vi "Status.Simple LED Status Indicator.vi"(7 "Show OK Indication":bool, 8 "error in":errorcluster, 10 "Blink on Error":bool, 11 "LED Status":refnum<vi>) -> (0 "error out":errorcluster)   [LabVIEW 2024, in "EQMF.lvlib" / "Status Utils.lvlib"]
uses:
  Status Utils.lvlib
panel:
  out "LED Status":bool
  in  "Test":bool
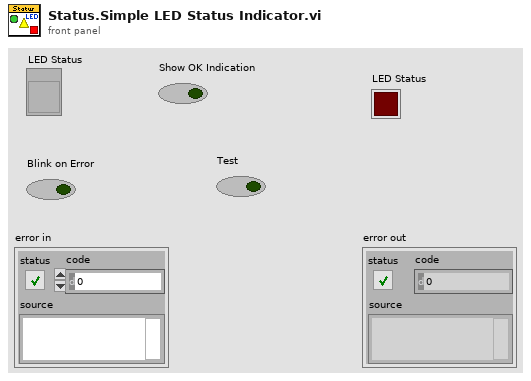
[diagram p1: front panel]
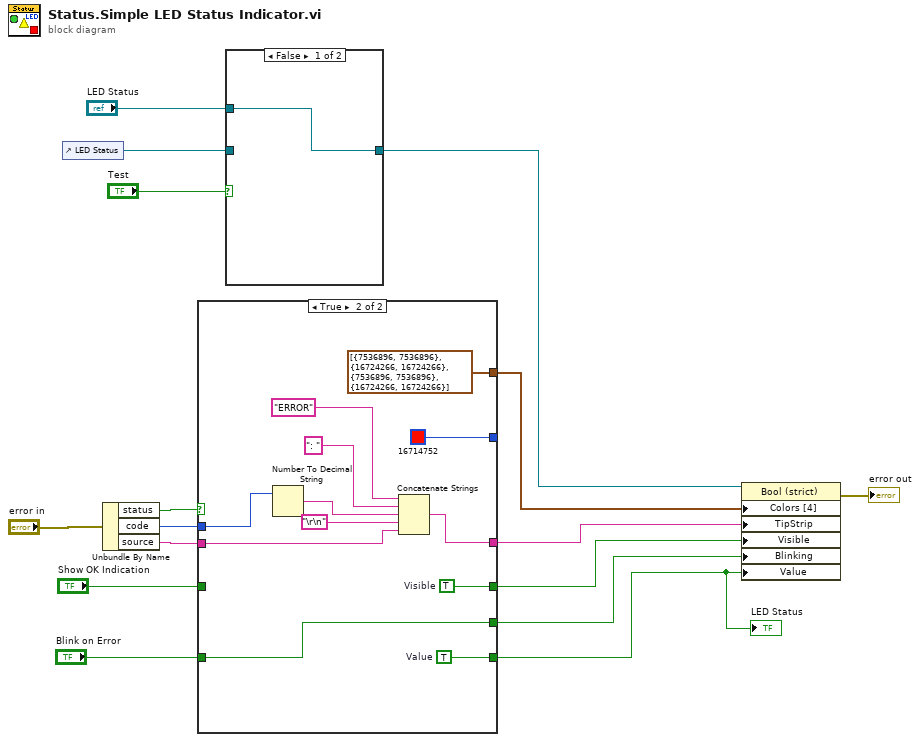
[diagram p0: block diagram]
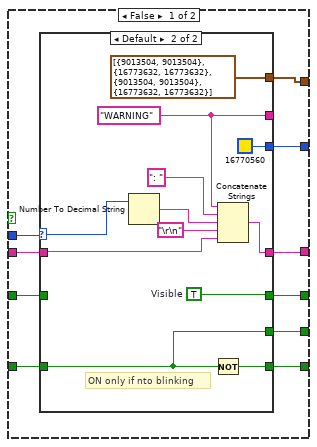
[diagram p2: hidden frame]
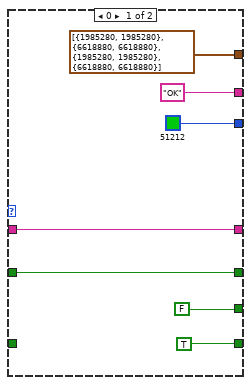
[diagram p3: hidden frame]
diagram:
  n1 = control-ref of="LED Status"() -> (w7:refnum<vi>)
  n2 = Unbundle By Name("error in") -> ("status"=w14:bool, "code"=w13:i32, "source"=w12:string)
  n3 = case shown="True" w14 {
    tunnel: w13 -> [w26 w56]
    tunnel: [w25 u32 16714752] -> _
    tunnel: w12 -> [w24 w53]
    tunnel: [w23 w52] -> w11
    tunnel: [w22 w49] -> w5
    tunnel: [w21 cluster{u32, u32}[] [{7536896, 7536896}, {16724266, 16724266}, {7536896, 7536896}, {16724266, 16724266}] ("Colors [4] 2")] -> w6
    tunnel: [w20 w46] -> w4
    tunnel: [w17 w47] -> w3
    tunnel: "Show OK Indication" -> [w19 _]
    tunnel: "Blink on Error" -> [w18 w46]
    frame False {
      n4 = case shown="Default" w26 {
        selector: w26 -> [_ w42]
        tunnel: [u32 51212 u32 16770560] -> w25
        tunnel: w24 -> [w32 w41]
        tunnel: [w32 w40] -> w23
        tunnel: ["OK" w38] -> _
        tunnel: [w29 w37] -> w22
        tunnel: [cluster{u32, u32}[] [{1985280, 1985280}, {6618880, 6618880}, {1985280, 1985280}, {6618880, 6618880}] ("Colors [4] 2") cluster{u32, u32}[] [{9013504, 9013504}, {16773632, 16773632}, {9013504, 9013504}, {16773632, 16773632}] ("Colors [4] 2")] -> w21
        tunnel: [FALSE w34] -> w20
        tunnel: [TRUE w35] -> w17
        tunnel: w19 -> [w29 _]
        tunnel: w18 -> [_ w34]
        frame 0 {
        }
        frame Default {
          w37 = TRUE  # Visible
          w38 = "WARNING"
          # "ON only if nto blinking"
          n5 = Number To Decimal String(number=w42) -> (decimal integer string=w44:string)  [unwired: 1 in]
          n6 = Not(x=w34) -> (.not. x?=w35:bool)
          n7 = Concatenate Strings(w38, ": ", w44, "\r\n", w41) -> (w40:string)
        }
      }
    }
    frame True {
      w47 = TRUE  # Value
      w49 = TRUE  # Visible
      n8 = Number To Decimal String(number=w56) -> (decimal integer string=w55:string)  [unwired: 1 in]
      n9 = Concatenate Strings("ERROR", ": ", w55, "\r\n", w53) -> (w52:string)
    }
  }
  "LED Status" <- w3
  n10 = case shown="False" "Test" {
    tunnel: "LED Status" -> [w58 _]
    tunnel: w7 -> [_ w59]
    tunnel: [w58 w59] -> w8
    frame False {
    }
    frame True {
    }
  }
  n11 = property on="Property Node" class="Bool (strict)"(reference=w8, "Colors [4]"=w6, "TipStrip"=w11, "Visible"=w5, "Blinking"=w4, "Value"=w3) -> (error out=→"error out":errorcluster)  [unwired: 1 in, 1 out]
